vi "Configure Modulation Input.vi"(8 "error in (no error)":errorcluster, 10 "Modulation Input (1: 5 V Level)":i32(ring)=1 items=["1 V Level", "5 V Level"], 11 "VISA resource name":refnum<visa-resource-name>) -> (0 "error out":errorcluster, 3 "VISA resource name out":refnum<visa-resource-name>)   [LabVIEW 2017, in "Agilent 3352X Series.lvlib"]
doc: "Specifies whether the modulation input on the 33600 Series works with signals up to the 5 V level or the 1 V level.\n\n<b>Note</b>:\n(1) This VI is only applicable for 33611A, 33612A, 33621A and 33622A models.\n(2) You can set this from the front panel modulation parameters screen if the modulation source is set to External."
uses:
  Doppia_Freq_Circuito/Agilent 3352X Series/Agilent 3352X Series.lvlib
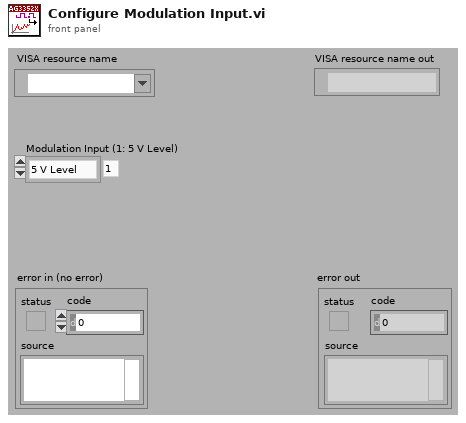
[diagram p1: front panel]
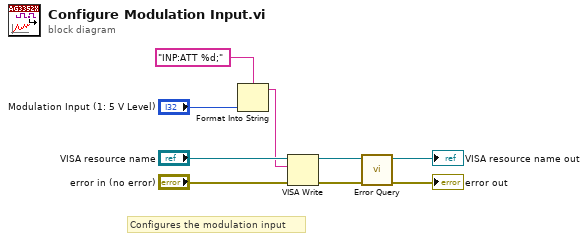
[diagram p0: block diagram]
diagram:
  # "Configures the modulation input"
  n1 = Format Into String(format string="INP:ATT %d;", "Modulation Input (1: 5 V Level)") -> (resulting string=w1:string)  [unwired: 2 in, 1 out]
  n2 = VISA Write(VISA resource name="VISA resource name", write buffer=w1, error in (no error)="error in (no error)") -> (VISA resource name out=w7:refnum<visa-resource-name>, error out=w6:errorcluster)  [unwired: 1 out]
  n3 = call "Error Query.vi"("error in (no error)"=w6, "VISA resource name"=w7) -> ("error out"=→"error out":errorcluster, "VISA resource name out"=→"VISA resource name out":refnum<visa-resource-name>)  [unwired: 8 out]
